vi "SetAdminPassword.vi"(8 "error in":errorcluster, 11 "New Password":string) -> (0 "error out":errorcluster)   [LabVIEW 2017]
uses:
  <vilib>/addons/InsightCM/Utilities/RT Images/InsightCM/brniauth.dll
panel:
  out "return type":i32
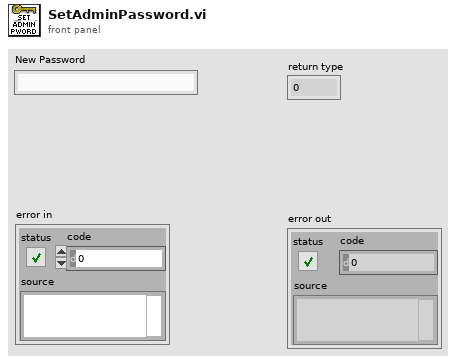
[diagram p1: front panel]
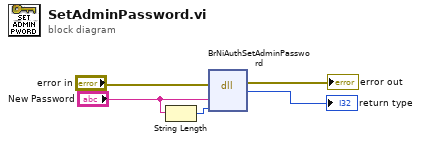
[diagram p0: block diagram]
diagram:
  n1 = String Length(string="New Password") -> (length=w4:i32)
  n2 = dll-call lib="C:/Program Files (x86)/National Instruments/LabVIEW 2017/vi.lib/addons/InsightCM/Utilities/RT Images/InsightCM/brniauth.*" fn="BrNiAuthSetAdminPassword"(error in="error in", "NewPassword"="New Password", "PasswordLength"=w4) -> (error out=→"error out":errorcluster, "return type"=→"return type":i32)  [unwired: 4 in, 1 out]
